vi "Post-Build Action.vi"(5 "Files Generated by Build":path[](array[path]), 6 "Top Level/Always Included VIs":path[](array[path]), 7 "Destination Path":path, 8 "Error In":errorcluster, 9 "Target Name":string, 10 "Build Specification Name":string, 11 "Project Path":path) -> (0 "Error Out":errorcluster)   [LabVIEW 2020]
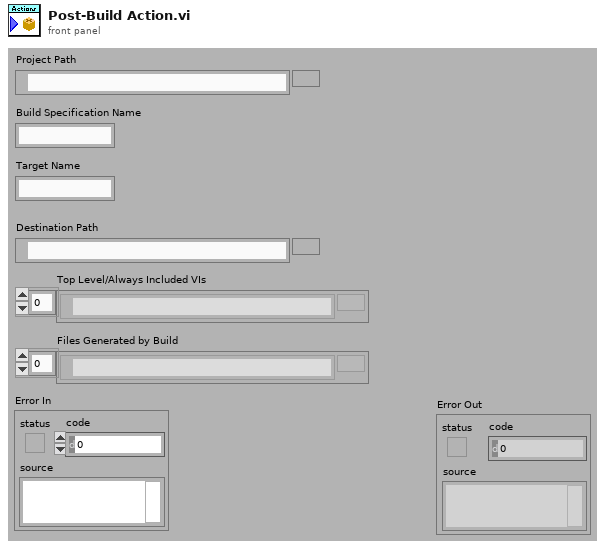
[diagram p1: front panel]
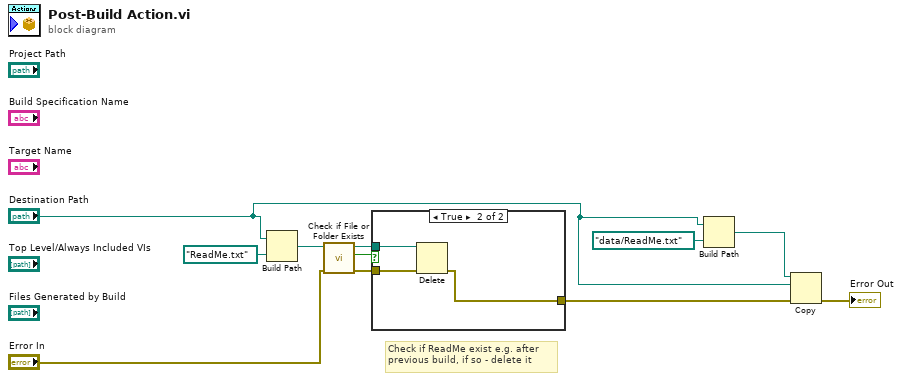
[diagram p0: block diagram]
diagram:
  # "Check if ReadMe exist e.g. after \nprevious build, if so - delete it"
  n1 = Build Path(base path="Destination Path", name or relative path=path "ReadMe.txt") -> (appended path=w7:path)
  n2 = call <vilib>:"Check if File or Folder Exists.vi"("error in (no error)"="Error In", "path"=w7) -> ("error out"=w5:errorcluster, "file or folder exists?"=w4:bool, "dup path"=w3:path)  [unwired: 7 in]
  n3 = case shown="True" w4 {
    tunnel: w5 -> [w12 w15]
    tunnel: w3 -> [_ w14]
    tunnel: [w12 w13] -> w2
    frame False {
    }
    frame True {
      n4 = Delete(path (use dialog)=w14, error in=w15) -> (error out=w13:errorcluster)  [unwired: 3 in, 2 out]
    }
  }
  n5 = Build Path(base path="Destination Path", name or relative path=path "data/ReadMe.txt") -> (appended path=w10:path)
  n6 = Copy(8:w2, 10:"Destination Path", 11:w10) -> (0:→"Error Out":errorcluster)  [unwired: 2 in, 2 out]
